vi "Remove Field UI.vi"(11 "Field Names":string[](array[string])) -> (2 "Cancelled":bool, 3 "Index":i32)   [LabVIEW 2020, in "Conditum-Tools.lvlib" / "Entity Editor.lvclass"]
uses:
  Entity Editor.lvclass
panel:
  in  "Cancel":bool
  in  "OK":bool
  in  "Field":i32(listbox)
  # "Select the field to remove:"
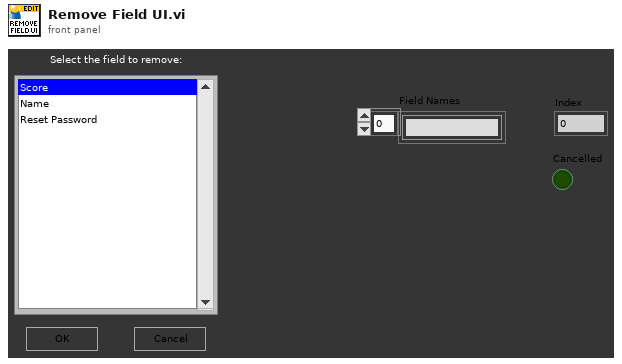
[diagram p1: front panel]
types:
  T1 = enum8{"Enabled", "Disabled", "Disabled and Grayed Out"}
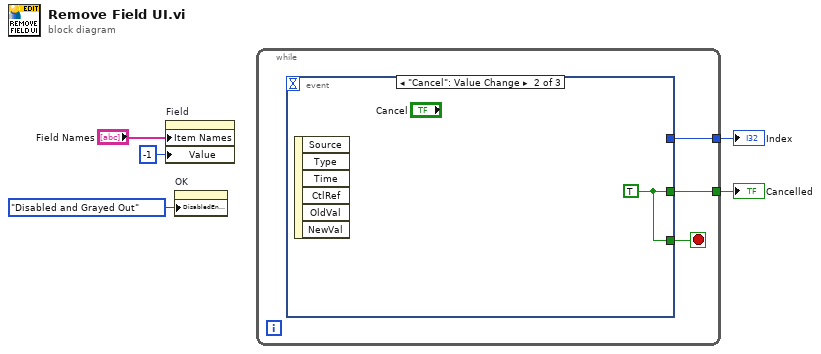
[diagram p0: block diagram]
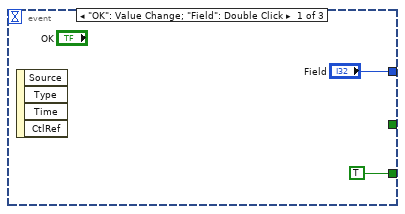
[diagram p2: hidden frame]
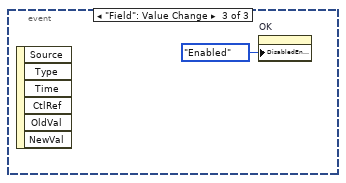
[diagram p3: hidden frame]
diagram:
  n1 = property on="Field" class="LstBox (strict)"("Item Names"="Field Names", "Value"=-1 ("Field")) -> ()  [unwired: 2 in, 2 out]
  n2 = property on="OK" class="Bool"("DisabledEnum"=T1."Disabled and Grayed Out" ("Disabled")) -> ()  [unwired: 2 in, 2 out]
  n3 = while {
    tunnel: [w7] -> w2
    tunnel: [w6] -> w1
    stop <- w8 stop-if-true
    n4 = event shown="[1] \"Cancel\": Value Change" {
      selector: _ -> [_ _ _]
      dyn-events: _ -> [_ _ _]
      timeout: _ -> [_ _ _]
      tunnel: [TRUE w11 _] -> w8
      tunnel: ["Field" _ _] -> w7
      tunnel: [_ w11 _] -> w6
      event "OK": Value Change; "Field": Double Click {
        n5 = event-data() -> ()  [unwired: 1 in, 4 out]
      }
      event "Cancel": Value Change {
        w11 = TRUE
        n6 = event-data() -> ()  [unwired: 1 in, 6 out]
      }
      event "Field": Value Change {
        n7 = event-data() -> ()  [unwired: 1 in, 6 out]
        n8 = property on="OK" class="Bool"("DisabledEnum"=T1."Enabled" ("Disabled")) -> ()  [unwired: 2 in, 2 out]
      }
    }
  }
  "Index" <- w2
  "Cancelled" <- w1
